vi "Power Read.vi"   [LabVIEW 2023, in "Power Supply.lvclass"]
uses:
  Power Supply.lvclass
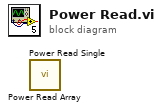
[diagram p0: block diagram]
diagram:
  n1 = call "Power Read Array.vi"() -> ()  [unwired: 9 in, 3 out]
  n2 = call "Power Read Single.vi"() -> ()  [unwired: 8 in, 4 out]
